vi "Update.vi"(8 "error in (no error)":errorcluster, 10 "BrowerComponent":refnum<class "BrowerComponent.lvclass">, 11 "BrowerGuidencer in":refnum<class "BrowerGuidencer.lvclass">) -> (0 "error out":errorcluster, 2 "BrowerComponent out":refnum<class "BrowerComponent.lvclass">, 3 "BrowerGuidencer out":refnum<class "BrowerGuidencer.lvclass">)   [LabVIEW 2015, in "BrowerGuidencer.lvclass"]
uses:
  BrowerGuidencer.lvclass
  BrowerComponent/BrowerComponent/BrowerComponent.lvclass
  BrowerGuidencer.lvclass/BrowerGuidencer.ctl
  AbstractBuilder/AbstractBuilder.lvclass
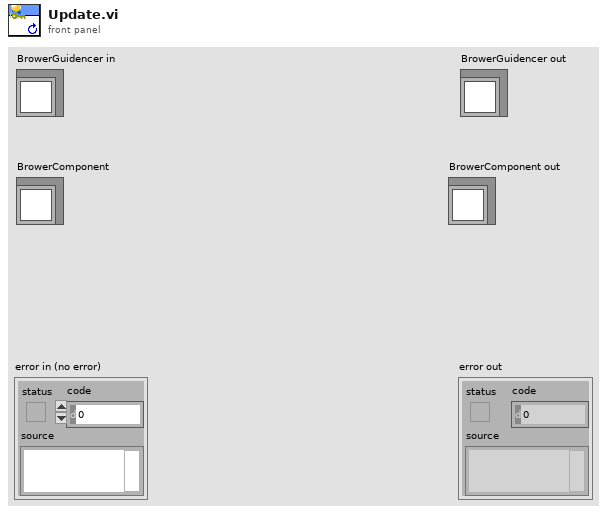
[diagram p1: front panel]
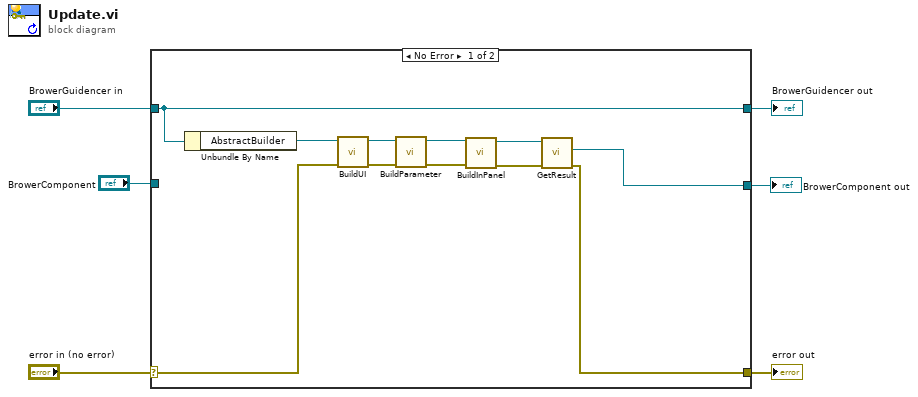
[diagram p0: block diagram]
diagram:
  n1 = case shown="No Error" "error in (no error)" {
    selector: "error in (no error)" -> [w15 w19]
    tunnel: [w7 w19] -> w5
    tunnel: [w17 w18] -> w3
    tunnel: "BrowerGuidencer in" -> [w17 w18]
    tunnel: "BrowerComponent" -> [_ _]
    tunnel: [w8 _] -> w1
    frame No Error {
      n2 = Unbundle By Name(w17) -> ("AbstractBuilder"=w16:refnum<class "AbstractBuilder.lvclass">)
      n3 = call-dynamic "BuildUI.vi"("error in (no error)"=w15, "reference in"=w16) -> ("error out"=w13:errorcluster, "reference out"=w14:refnum<class "AbstractBuilder.lvclass">)  [unwired: 8 in]
      n4 = call-dynamic "BuildParameter.vi"("error in (no error)"=w13, "AbstractBuilder in"=w14) -> ("error out"=w11:errorcluster, "AbstractBuilder out"=w12:refnum<class "AbstractBuilder.lvclass">)  [unwired: 8 in]
      n5 = call-dynamic "BuildInPanel.vi"("error in (no error)"=w11, "AbstractBuilder in"=w12) -> ("error out"=w9:errorcluster, "AbstractBuilder out"=w10:refnum<class "AbstractBuilder.lvclass">)  [unwired: 8 in]
      n6 = call-dynamic "GetResult.vi"("error in (no error)"=w9, "AbstractBuilder in"=w10) -> ("error out"=w7:errorcluster, "BrowerComponent"=w8:refnum<class "BrowerComponent.lvclass">)  [unwired: 7 in, 1 out]
    }
    frame Error {
    }
  }
  "error out" <- w5
  "BrowerGuidencer out" <- w3
  "BrowerComponent out" <- w1
